vi "ClearLists.vi"(8 "error in (no error)":errorcluster, 11 "UI Refs":T1) -> (0 "error out":errorcluster, 3 "UI Refs":T1)   [LabVIEW 2015]
uses:
  Controls & Type Defs/UI Data.ctl
  <vilib>/Utility/miscctls.llb/LVRowAndColumnUnsignedTypeDef.ctl
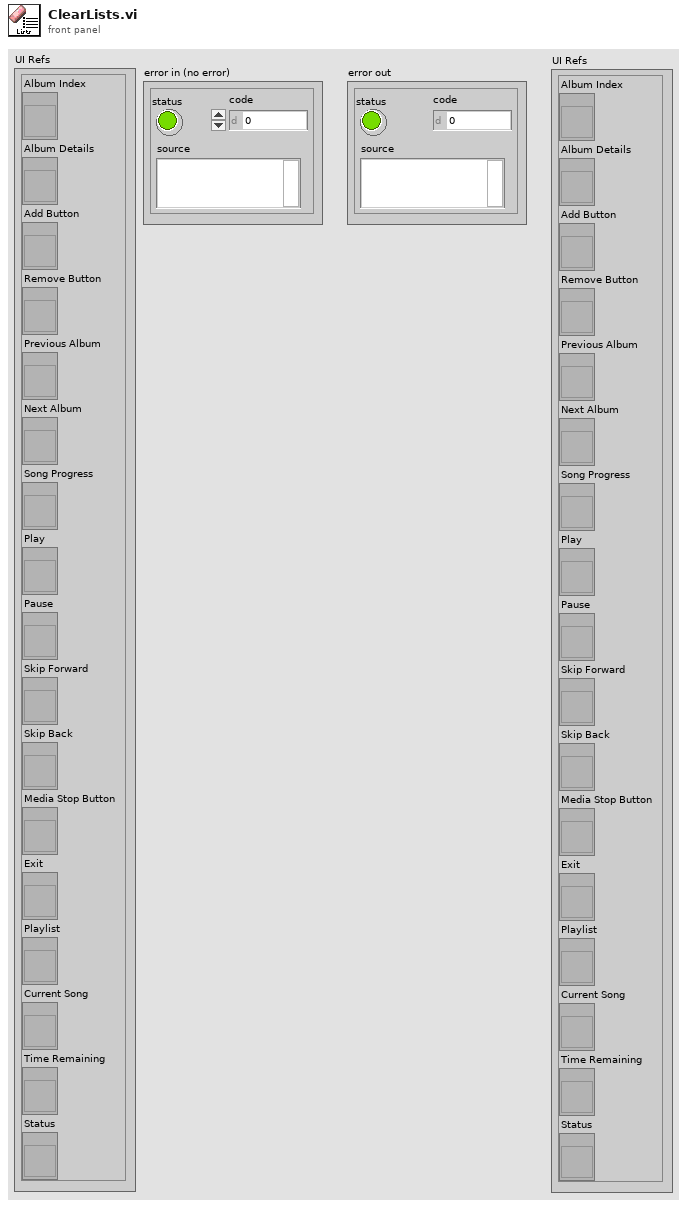
[diagram p1: front panel]
types:
  T1 = typedef "UI Data.ctl" = cluster{"Album Index":refnum<vi>, "Album Details":refnum<vi>, "Add Button":refnum<vi>, "Remove Button":refnum<vi>, "Previous Album":refnum<vi>, "Next Album":refnum<vi>, "Song Progress":refnum<vi>, "Play":refnum<vi>, "Pause ":refnum<vi>, "Skip Forward":refnum<vi>, "Skip Back":refnum<vi>, "Media Stop Button":refnum<vi>, "Exit":refnum<vi>, "Playlist":refnum<vi>, "Current Song":refnum<vi>, "Time Remaining":refnum<vi>, "Status":refnum<vi>}
  T2 = typedef "LVRowAndColumnUnsignedTypeDef.ctl" = cluster{"Row":u32, "Column":u32}
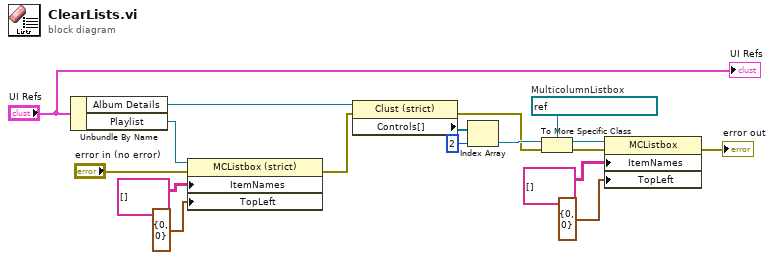
[diagram p0: block diagram]
diagram:
  w8 = refnum<vi> refnum  # MulticolumnListbox
  n1 = Unbundle By Name("UI Refs") -> ("Album Details"=w13:refnum<vi>, "Playlist"=w14:refnum<vi>)
  n2 = property class="MCListbox (strict)"(reference=w14, error in="error in (no error)", "ItemNames"=string[][] [] ("Item Names"), "TopLeft"=T2 {"Row"=0, "Column"=0} ("Top Left Visible Cell")) -> (error out=w9:errorcluster)  [unwired: 1 out]
  n3 = property class="Clust (strict)"(reference=w13, error in=w9) -> (error out=w10:errorcluster, "Controls[]"=w12:refnum<vi>[])  [unwired: 1 out]
  n4 = Index Array(array=w12, index=2) -> (element=w11:refnum<vi>)
  n5 = To More Specific Class(target class=w8, reference=w11, error in=w10) -> (specific class reference=w7:refnum<vi>, error out=w6:errorcluster)
  n6 = property class="MCListbox"(reference=w7, error in=w6, "ItemNames"=string[][] [] ("Item Names"), "TopLeft"=T2 {"Row"=0, "Column"=0} ("Top Left Visible Cell")) -> (error out=→"error out":errorcluster)  [unwired: 1 out]
  "UI Refs" <- "UI Refs"
